vi "StrainTestCell3.vi"() -> ()   [LabVIEW 2020]
uses:
  <instrlib>/NH Research Regenerative Test Series/Public/Configure/Output Safety.ctl
  Readings.vi
  <instrlib>/NH Research Regenerative Test Series/Public/Data/Read (Ave Current).vi
  <instrlib>/NH Research Regenerative Test Series/Public/Data/Low Level/Fetch (Ave Voltage).vi
  <instrlib>/NH Research Regenerative Test Series/Public/Data/Low Level/Fetch (Ave True Power).vi
  <instrlib>/NH Research Regenerative Test Series/Public/Data/Read (Ave Voltage).vi
  <instrlib>/NH Research Regenerative Test Series/NH Research Regenerative Test Series.lvlib
panel:
  in  "Current Cutoff 2":dbl
  in  "Discharge Folder Path":path
  out "Charge Strain":dbl(graph)
  out "Discharge Strain":dbl(graph)
  in  "DWaitStop":bool
  out "Discharge Rest":bool
  in  "Wait Time":u32
  out "Elaspsed Time":u32 caption="Elapsed Time (s)"
  in  "CWait Stop":bool
  out "Charge Rest":bool
  in  "Wait Time":u32
  out "Elapsed Time":u32 caption="Elapsed Time (s)"
  out "Discharge Rest Voltage":dbl
  out "Charge Rest Voltage":dbl
  in  "1C Preset 2":bool
  out "Discharging":bool
  in  "Discharge Stop":bool
  in  "Discharge Current":dbl
  in  "Voltage Cutoff":dbl
  in  "1C Preset":bool
  out "Strain":dbl
  out "Ave Current (A)":dbl
  out "Ave Voltage (V)":dbl
  out "Ave True Power (W)":dbl
  out "Battemp":dbl
  out "AmbientTemp":dbl
  out "Discharge Rest Voltage":dbl(graph)
  out "Charge Rest Voltage":dbl(graph)
  in  "Tab Control":T1(tab)
  out "Selected Output Safety":T2
  in  "Custom Output Safety":T2
  in  "Output Safety\nSelection":bool caption="Output Safety"
  in  "Charge Folder Path":path
  in  "Cell Number":string
  in  "DAQmx Task Name":refnum<k21>
  in  "NHR VISA Name":refnum<visa-resource-name>
  out "Error Out":string
  out "Previous Discharge Data File":path caption="Filename Out"
  out "File Name":path caption="Filename Out"
  out "D Wait Status Byte Register":T3
  out "Discharge Status Byte Register":T3
  out "C Wait Status Byte Register":T3
  out "Charge Status Byte Register":T3
  out "Task error out":errorcluster
  in  "Cycle Stop":bool
  out "Cycle Index":i32
  in  "Number of Cycles":i32
  out "Charging":bool
  in  "Charge Stop":bool
  in  "Current Cutoff":dbl
  in  "Charge Current":dbl format="%#.6g"
  in  "Charge Voltage":dbl format="%#.6g"
  out "Tab Control 2":T1(tab)
  in  "Logical Instrument Number":u32=1
  # "Readings"
  # "Cycle & Charge Profile Settings"
  # "Charging"
  # "Discharging"
  # "Post Charge\nRest"
  # "Post Discharge\nRest"
  # "Cycle\nInfo"
  # "Rest Voltage Charts"
  # "Output Safety Configuration"
  # "Test Name & Device Info"
  # "Error Indication"
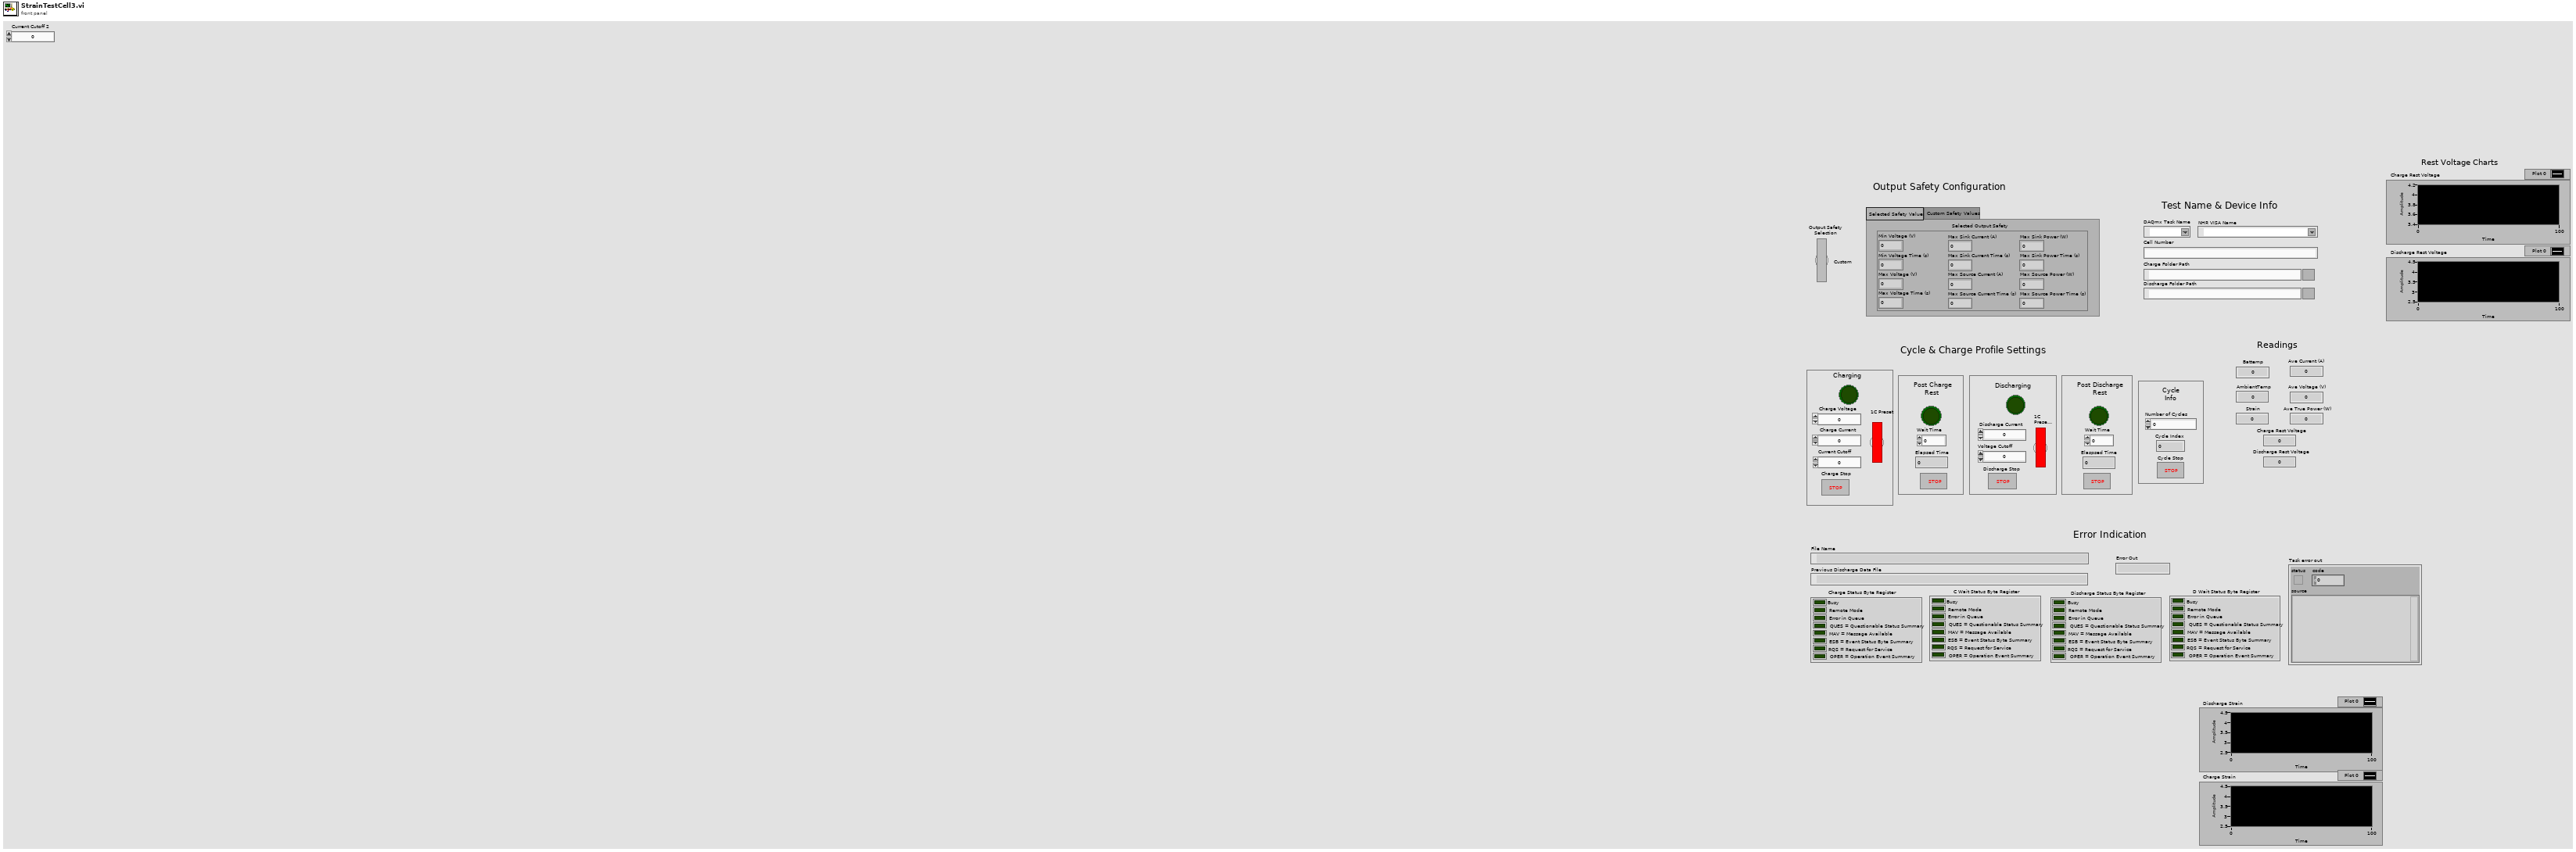
[diagram p1: front panel]
types:
  T1 = enum32{"Selected Safety Values", "Custom Safety Values"}
  T2 = typedef "NH Research Regenerative Test Series.lvlib/Output Safety.ctl" = cluster{"Min Voltage (V)":dbl, "Min Voltage Time (s)":dbl, "Max Voltage (V)":dbl, "Max Voltage Time (s)":dbl, "Max Sink Current (A)":dbl, "Max Sink Current Time (s)":dbl, "Max Source Current (A)":dbl, "Max Source Current Time (s)":dbl, "Max Sink Power (W)":dbl, "Max Sink Power Time (s)":dbl, "Max Source Power (W)":dbl, "Max Source Power Time (s)":dbl}
  T3 = cluster{"Busy":bool, "Remote Mode":bool, "Error in Queue":bool, "QUES = Questionable Status Summary":bool, "MAV = Message Available":bool, "ESB = Event Status Byte Summary":bool, "RQS = Request for Service":bool, "OPER = Operation Event Summary":bool}
  T4 = cluster{"Min Voltage (V)":dbl, "Min Voltage Time (s)":dbl, "Max Voltage (V)":dbl, "Max Voltage Time (s)":dbl, "Max Sink Current (A)":dbl, "Max Sink Current Time (s)":dbl, "Max Source Current (A)":dbl, "Max Source Current Time (s)":dbl, "Max Sink Power (W)":dbl, "Max Sink Power Time (s)":dbl, "Max Source Power (W)":dbl, "Max Source Power Time (s)":dbl}
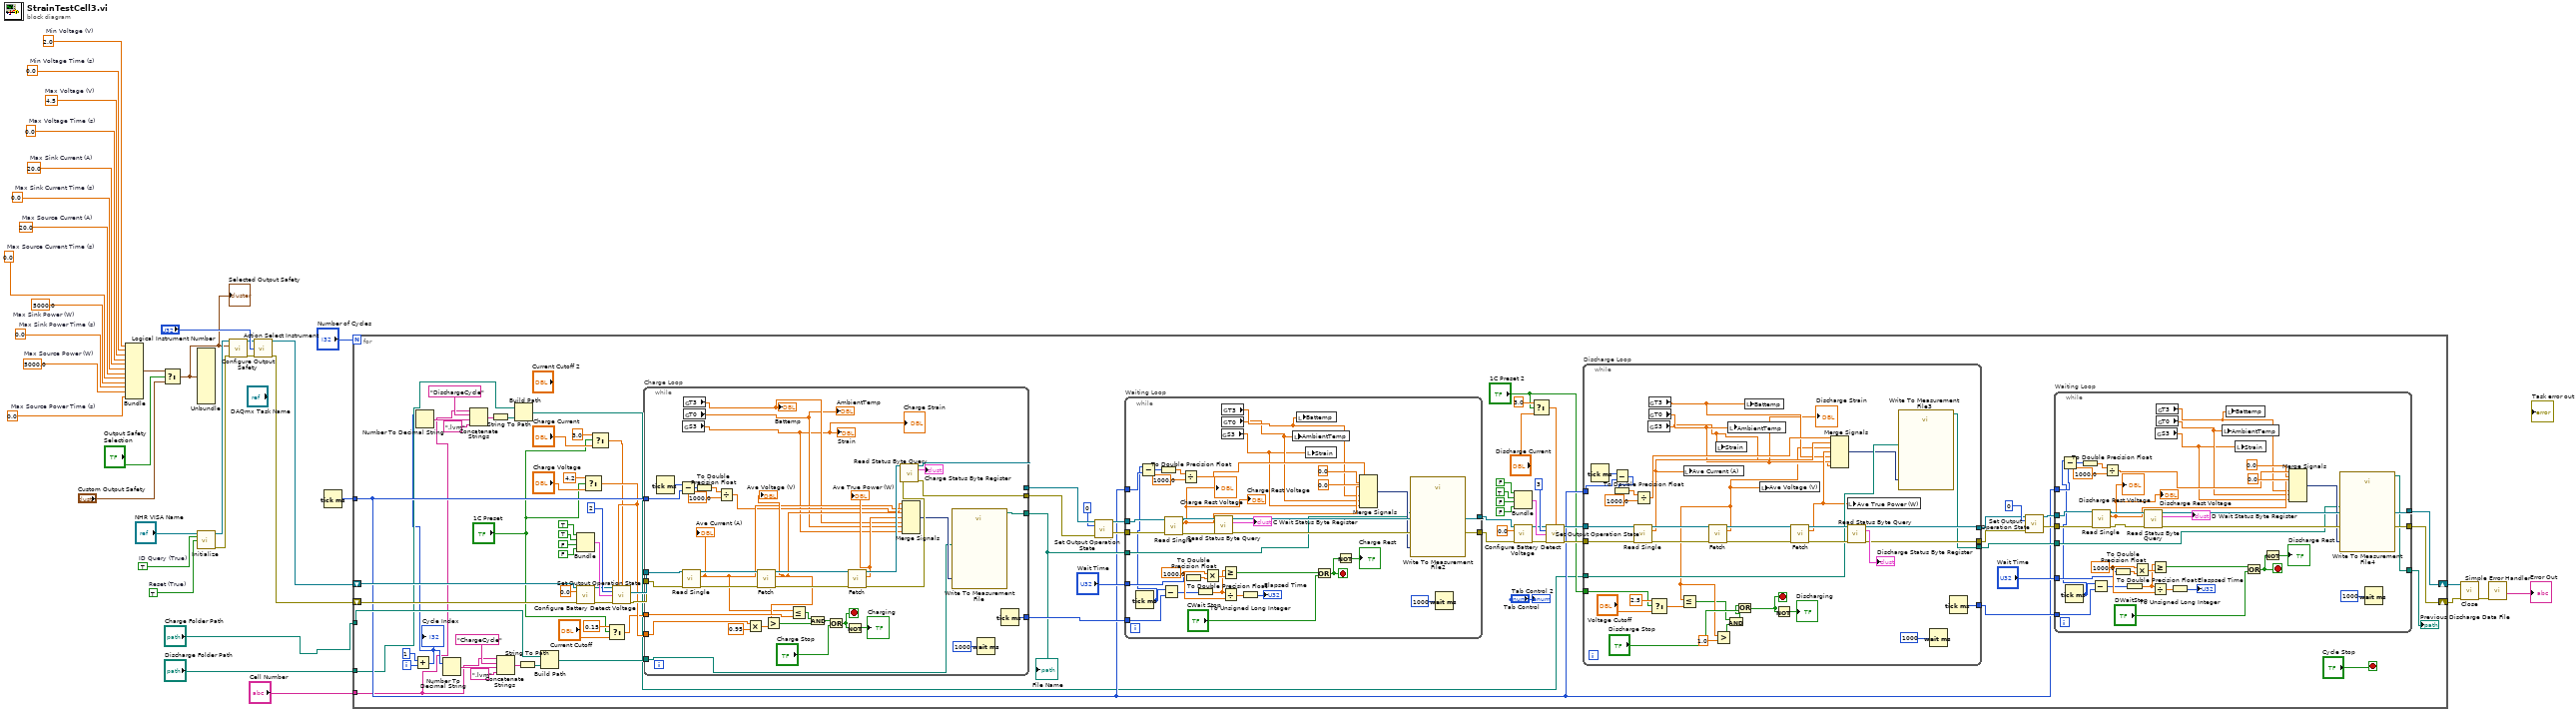
[diagram p0: block diagram]
diagram:
  w10 = 5000.0  # Max Source Power (W)
  w11 = 0.0  # Max Sink Power Time (s)
  w12 = 5000.0  # Max Sink Power (W)
  w13 = 0.0  # Max Source Current Time (s)
  w14 = 20.0  # Max Source Current (A)
  w16 = 20.0  # Max Sink Current (A)
  w15 = 0.0  # Max Sink Current Time (s)
  w17 = 0.0  # Max Voltage Time (s)
  w18 = 4.5  # Max Voltage (V)
  w19 = 2.0  # Min Voltage (V)
  w9 = 0.0  # Max Source Power Time (s)
  w20 = 0.0  # Min Voltage Time (s)
  w34 = TRUE  # ID Query (True)
  w33 = TRUE  # Reset (True)
  n1 = Bundle("Min Voltage (V)"=w19, "Min Voltage Time (s)"=w20, "Max Voltage (V)"=w18, "Max Voltage Time (s)"=w17, "Max Sink Current (A)"=w16, "Max Sink Current Time (s)"=w15, "Max Source Current (A)"=w14, "Max Source Current Time (s)"=w13, "Max Sink Power (W)"=w12, "Max Sink Power Time (s)"=w11, "Max Source Power (W)"=w10, "Max Source Power Time (s)"=w9) -> (w7:T4)  [unwired: 1 in]
  n2 = Select(t=w7, s="Output Safety\nSelection", f="Custom Output Safety") -> (s? t:f=w8:T2)
  "Selected Output Safety" <- w8
  n3 = Unbundle(w8) -> ()  [unwired: 12 out]
  n4 = call <vilib>:"Initialize.vi"("VISA resource name"="NHR VISA Name", "ID Query (True)"=w34, "Reset (True)"=w33) -> ("VISA resource name out"=w32:refnum<visa-resource-name>, "error out"=w31:errorcluster)  [unwired: 11 in]
  n5 = call <vilib>:"Configure Output Safety.vi"("VISA resource name"=w32, "Output Safety"=w8, "error in (no error)"=w31) -> ("VISA resource name out"=w29:refnum<visa-resource-name>, "error out"=w28:errorcluster)  [unwired: 11 in]
  n6 = call <instrlib>:"Action Select Instrument.vi"("VISA resource name"=w29, "Logical Instrument Number"="Logical Instrument Number", "error in (no error)"=w28) -> ("VISA resource name out"=w25:refnum<visa-resource-name>, "error out"=w24:errorcluster)  [unwired: 11 in]
  n7 = Tick Count (ms)() -> (millisecond timer value=w4:u32)
  n8 = for {
    N: "Number of Cycles" -> [_]
    shift-right: [w63] -> w23
    shift-left: w25 -> [w91]
    shift-right: [w62] -> w22
    shift-left: w24 -> [w89]
    tunnel: "Charge Folder Path" -> [w60]
    tunnel: w4 -> [w59]
    tunnel: "Cell Number" -> [w37]
    tunnel: "Discharge Folder Path" -> [w39]
    i -> [w86]
    stop <- "Cycle Stop" stop-if-true
    n9 = Add(x=1, y=w86) -> (x+y=w38:i32)
    "Cycle Index" <- w38
    n10 = Number To Decimal String(number=w38) -> (decimal integer string=w41:string)  [unwired: 1 in]
    n11 = Number To Decimal String(number=w38) -> (decimal integer string=w76:string)  [unwired: 1 in]
    n12 = Concatenate Strings(w37, "DischargeCycle", w41, ".lvm") -> (w42:string)
    n13 = String To Path(string=w42) -> (path=w43:path)
    n14 = Concatenate Strings(w37, "ChargeCycle", w76, ".lvm") -> (w81:string)
    n15 = Build Path(base path=w39, name or relative path=w43) -> (appended path=w36:path)
    n16 = String To Path(string=w81) -> (path=w82:path)
    n17 = Build Path(base path=w60, name or relative path=w82) -> (appended path=w78:path)
    n18 = Bundle(TRUE, TRUE, FALSE, FALSE) -> (w92:cluster{bool, bool, bool, bool})  [unwired: 1 in]
    n19 = call <vilib>:"Configure Battery Detect Voltage.vi"("VISA resource name"=w91, "Battery Detect Voltage (0V)"=0.0, "error in (no error)"=w89) -> ("VISA resource name out"=w90:refnum<visa-resource-name>, "error out"=w88:errorcluster)  [unwired: 11 in]
    n20 = Select(t=4.2, s="1C Preset", f="Charge Voltage") -> (s? t:f=w56:dbl)
    n21 = Select(t=3.0, s="1C Preset", f="Charge Current") -> (s? t:f=w55:dbl)
    n22 = Select(t=0.15, s="1C Preset", f="Current Cutoff") -> (s? t:f=w51:dbl)
    n23 = call <vilib>:"Set Output Operation State.vi"("VISA resource name"=w90, "Voltage Setpoint (0 V)"=w56, "Current Setpoint (0 A)"=w55, "Mode (0: Off)"=2, "Enable"=w92, "error in (no error)"=w88) -> ("VISA resource name out"=w98:refnum<visa-resource-name>, "error out"=w97:errorcluster)  [unwired: 8 in]
    n24 = while "Charge Loop" {
      tunnel: w98 -> [w257]
      tunnel: w97 -> [w256]
      tunnel: [w254] -> w103
      tunnel: [w253] -> w102
      tunnel: w51 -> [w249]
      tunnel: w78 -> [w244]
      tunnel: [w250] -> w72
      tunnel: [w245] -> w85
      tunnel: w56 -> [w236]
      tunnel: w59 -> [w234]
      stop <- w241 stop-if-true
      n25 = Tick Count (ms)() -> (millisecond timer value=w235:u32)
      n26 = Subtract(x=w235, y=w234) -> (x-y=w233:u32)
      n27 = call-poly <instrlib>:"Read Single.vi"("VISA resource name"=w257, "error in (no error)"=w256) -> ("VISA resource name out"=w262:refnum<visa-resource-name>, "Ave Current (A)"=w230:dbl, "error out"=w263:errorcluster)  [unwired: 11 in]
      "Ave Current (A)" <- w230
      n28 = global read "Readings.vi" "S3"() -> (w226:dbl)
      "Strain" <- w226
      "Charge Strain" <- w226
      n29 = global read "Readings.vi" "T3"() -> (w228:dbl)
      "Battemp" <- w228
      n30 = global read "Readings.vi" "T0"() -> (w227:dbl)
      "AmbientTemp" <- w227
      n31 = To Double Precision Float(number=w233) -> (double precision float=w231:dbl)
      n32 = Divide(x=w231, y=1000.0) -> (x/y=w229:dbl)
      n33 = Multiply(x=w236, y=0.95) -> (x*y=w238:dbl)
      n34 = call-poly <instrlib>:"Fetch.vi"("VISA resource name"=w262, "error in (no error)"=w263) -> ("VISA resource name out"=w261:refnum<visa-resource-name>, "Ave Voltage (V)"=w239:dbl, "error out"=w260:errorcluster)  [unwired: 11 in]
      "Ave Voltage (V)" <- w239
      n35 = Greater?(x=w239, y=w238) -> (0:w246:bool)
      n36 = Less Or Equal?(x=w230, y=w249) -> (x <= y?=w247:bool)
      n37 = And(x=w247, y=w246) -> (x .and. y?=w243:bool)
      n38 = Or(x=w243, y="Charge Stop") -> (x .or. y?=w241:bool)
      n39 = Not(x=w241) -> (.not. x?=→"Charging":bool)
      n40 = call-poly <instrlib>:"Fetch.vi"("VISA resource name"=w261, "error in (no error)"=w260) -> ("VISA resource name out"=w259:refnum<visa-resource-name>, "Ave True Power (W)"=w252:dbl, "error out"=w258:errorcluster)  [unwired: 11 in]
      "Ave True Power (W)" <- w252
      n41 = call <instrlib>:"Read Status Byte Query.vi"("VISA resource name"=w259, "error in (no error)"=w258) -> ("VISA resource name out"=w254:refnum<visa-resource-name>, "Status Byte Register"=→"Charge Status Byte Register":T3, "error out"=w253:errorcluster)  [unwired: 11 in]
      n42 = Merge Signals "Merge Signals"(w229, w230, w239, w252, w228, w227, w226) -> (w251:dynamicdata)
      n43 = call "Write To Measurement File"("Signals"=w251, "Filename"=w244) -> ("Filename Out"=w250:path)  [unwired: 15 in, 2 out]
      n44 = Wait (ms)(milliseconds to wait=u32 1000) -> ()  [unwired: 1 out]
      n45 = Tick Count (ms)() -> (millisecond timer value=w245:u32)
    }
    "File Name" <- w72
    n46 = call <vilib>:"Set Output Operation State.vi"("VISA resource name"=w103, "Mode (0: Off)"=0, "error in (no error)"=w102) -> ("VISA resource name out"=w100:refnum<visa-resource-name>, "error out"=w74:errorcluster)  [unwired: 11 in]
    n47 = while "Waiting Loop" {
      tunnel: [w224] -> w105
      tunnel: "Wait Time" -> [w214]
      tunnel: w85 -> [w221]
      tunnel: w100 -> [w205]
      tunnel: w74 -> [w204]
      tunnel: [w212] -> w73
      tunnel: w72 -> [w209]
      tunnel: w59 -> [w203]
      stop <- w194 stop-if-true
      w222 = 1000.0
      n48 = Tick Count (ms)() -> (millisecond timer value=w202:u32)
      n49 = Subtract(x=w202, y=w203) -> (x-y=w199:u32)
      n50 = To Double Precision Float(number=w199) -> (double precision float=w200:dbl)
      n51 = Subtract(x=w202, y=w221) -> (x-y=w216:u32)
      n52 = call-poly <instrlib>:"Read Single.vi"("VISA resource name"=w205, "error in (no error)"=w204) -> ("VISA resource name out"=w207:refnum<visa-resource-name>, "Ave Voltage (V)"=w206:dbl, "error out"=w208:errorcluster)  [unwired: 11 in]
      "Charge Rest Voltage" <- w206
      "Charge Rest Voltage" <- w206
      n53 = Divide(x=w200, y=1000.0) -> (x/y=w197:dbl)
      n54 = To Double Precision Float(number=w214) -> (double precision float=w213:dbl)
      n55 = To Double Precision Float(number=w216) -> (double precision float=w215:dbl)
      n56 = Multiply(x=w222, y=w213) -> (x*y=w223:dbl)
      n57 = call <instrlib>:"Read Status Byte Query.vi"("VISA resource name"=w207, "error in (no error)"=w208) -> ("VISA resource name out"=w224:refnum<visa-resource-name>, "Status Byte Register"=→"C Wait Status Byte Register":T3, "error out"=w212:errorcluster)  [unwired: 11 in]
      n58 = global read "Readings.vi" "S3"() -> (w191:dbl)
      n59 = global read "Readings.vi" "T3"() -> (w193:dbl)
      n60 = global read "Readings.vi" "T0"() -> (w192:dbl)
      n61 = Greater Or Equal?(x=w215, y=w223) -> (x >= y?=w196:bool)
      n62 = Divide(x=w215, y=w222) -> (x/y=w218:dbl)
      n63 = To Unsigned Long Integer(number=w218) -> (unsigned 32bit integer=→"Elapsed Time":u32)
      n64 = local write "AmbientTemp"(w192) -> ()
      n65 = local write "Battemp"(w193) -> ()
      n66 = local write "Strain"(w191) -> ()
      n67 = Or(x=w196, y="CWait Stop") -> (x .or. y?=w194:bool)
      n68 = Not(x=w194) -> (.not. x?=→"Charge Rest":bool)
      n69 = Merge Signals "Merge Signals"(w197, 0.0, w206, 0.0, w193, w192, w191) -> (w210:dynamicdata)
      n70 = call "Write To Measurement File2"("Signals"=w210, "Filename"=w209) -> ()  [unwired: 15 in, 3 out]
      n71 = Wait (ms)(milliseconds to wait=u32 1000) -> ()  [unwired: 1 out]
    }
    n72 = Bundle(FALSE, TRUE, FALSE, FALSE) -> (w107:cluster{bool, bool, bool, bool})  [unwired: 1 in]
    n73 = call <vilib>:"Configure Battery Detect Voltage.vi"("VISA resource name"=w105, "Battery Detect Voltage (0V)"=0.0, "error in (no error)"=w73) -> ("VISA resource name out"=w104:refnum<visa-resource-name>, "error out"=w106:errorcluster)  [unwired: 11 in]
    n74 = Select(t=3.0, s="1C Preset 2", f="Discharge Current") -> (s? t:f=w46:dbl)
    n75 = call <vilib>:"Set Output Operation State.vi"("VISA resource name"=w104, "Current Setpoint (0 A)"=w46, "Mode (0: Off)"=3, "Enable"=w107, "error in (no error)"=w106) -> ("VISA resource name out"=w112:refnum<visa-resource-name>, "error out"=w113:errorcluster)  [unwired: 9 in]
    n76 = while "Discharge Loop" {
      tunnel: w112 -> [w184]
      tunnel: w113 -> [w183]
      tunnel: [w181] -> w67
      tunnel: [w180] -> w68
      tunnel: w36 -> [w179]
      tunnel: [w169] -> w66
      tunnel: [w172] -> w65
      tunnel: w59 -> [w170]
      tunnel: "1C Preset 2" -> [w160]
      stop <- w174 stop-if-true
      n77 = Tick Count (ms)() -> (millisecond timer value=w171:u32)
      n78 = Subtract(x=w171, y=w170) -> (x-y=w166:u32)
      n79 = To Double Precision Float(number=w166) -> (double precision float=w167:dbl)
      n80 = call-poly <instrlib>:"Read Single.vi"("VISA resource name"=w184, "error in (no error)"=w183) -> ("VISA resource name out"=w189:refnum<visa-resource-name>, "Ave Current (A)"=w165:dbl, "error out"=w190:errorcluster)  [unwired: 11 in]
      n81 = Divide(x=w167, y=1000.0) -> (x/y=w164:dbl)
      n82 = global read "Readings.vi" "S3"() -> (w157:dbl)
      "Discharge Strain" <- w157
      n83 = global read "Readings.vi" "T3"() -> (w159:dbl)
      n84 = global read "Readings.vi" "T0"() -> (w158:dbl)
      n85 = Select(t=2.5, s=w160, f="Voltage Cutoff") -> (s? t:f=w161:dbl)
      n86 = local write "Ave Current (A)"(w165) -> ()
      n87 = call-poly <instrlib>:"Fetch.vi"("VISA resource name"=w189, "error in (no error)"=w190) -> ("VISA resource name out"=w188:refnum<visa-resource-name>, "Ave Voltage (V)"=w155:dbl, "error out"=w187:errorcluster)  [unwired: 11 in]
      n88 = Less Or Equal?(x=w155, y=w161) -> (x <= y?=w152:bool)
      n89 = Greater?(x=w155, y=1.0) -> (0:w154:bool)
      n90 = local write "Strain"(w157) -> ()
      n91 = And(x=w152, y=w154) -> (x .and. y?=w153:bool)
      n92 = local write "AmbientTemp"(w158) -> ()
      n93 = Or(x=w153, y="Discharge Stop") -> (x .or. y?=w174:bool)
      n94 = local write "Battemp"(w159) -> ()
      n95 = local write "Ave Voltage (V)"(w155) -> ()
      n96 = Not(x=w174) -> (.not. x?=→"Discharging":bool)
      n97 = call-poly <instrlib>:"Fetch.vi"("VISA resource name"=w188, "error in (no error)"=w187) -> ("VISA resource name out"=w186:refnum<visa-resource-name>, "Ave True Power (W)"=w173:dbl, "error out"=w185:errorcluster)  [unwired: 11 in]
      n98 = Merge Signals "Merge Signals"(w164, w165, w155, w173, w159, w158, w157) -> (w178:dynamicdata)
      n99 = local write "Ave True Power (W)"(w173) -> ()
      n100 = call <instrlib>:"Read Status Byte Query.vi"("VISA resource name"=w186, "error in (no error)"=w185) -> ("VISA resource name out"=w181:refnum<visa-resource-name>, "Status Byte Register"=→"Discharge Status Byte Register":T3, "error out"=w180:errorcluster)  [unwired: 11 in]
      n101 = call "Write To Measurement File3"("Signals"=w178, "Filename"=w179) -> ("Filename Out"=w172:path)  [unwired: 15 in, 2 out]
      n102 = Wait (ms)(milliseconds to wait=u32 1000) -> ()  [unwired: 1 out]
      n103 = Tick Count (ms)() -> (millisecond timer value=w169:u32)
    }
    n104 = call <vilib>:"Set Output Operation State.vi"("VISA resource name"=w67, "Mode (0: Off)"=0, "error in (no error)"=w68) -> ("VISA resource name out"=w71:refnum<visa-resource-name>, "error out"=w70:errorcluster)  [unwired: 11 in]
    n105 = while "Waiting Loop" {
      tunnel: [w151] -> w63
      tunnel: "Wait Time" -> [w143]
      tunnel: w66 -> [w148]
      tunnel: w71 -> [w133]
      tunnel: w70 -> [w132]
      tunnel: [w141] -> w62
      tunnel: [w138] -> w61
      tunnel: w65 -> [w137]
      tunnel: w59 -> [w128]
      stop <- w119 stop-if-true
      w149 = 1000.0
      n106 = Tick Count (ms)() -> (millisecond timer value=w127:u32)
      n107 = Subtract(x=w127, y=w128) -> (x-y=w124:u32)
      n108 = To Double Precision Float(number=w124) -> (double precision float=w125:dbl)
      n109 = Subtract(x=w127, y=w148) -> (x-y=w145:u32)
      n110 = call-poly <instrlib>:"Read Single.vi"("VISA resource name"=w133, "error in (no error)"=w132) -> ("VISA resource name out"=w131:refnum<visa-resource-name>, "Ave Voltage (V)"=w130:dbl, "error out"=w129:errorcluster)  [unwired: 11 in]
      "Discharge Rest Voltage" <- w130
      "Discharge Rest Voltage" <- w130
      n111 = Divide(x=w125, y=1000.0) -> (x/y=w123:dbl)
      n112 = To Double Precision Float(number=w143) -> (double precision float=w142:dbl)
      n113 = To Double Precision Float(number=w145) -> (double precision float=w144:dbl)
      n114 = Multiply(x=w149, y=w142) -> (x*y=w150:dbl)
      n115 = call <instrlib>:"Read Status Byte Query.vi"("VISA resource name"=w131, "error in (no error)"=w129) -> ("VISA resource name out"=w151:refnum<visa-resource-name>, "Status Byte Register"=→"D Wait Status Byte Register":T3, "error out"=w141:errorcluster)  [unwired: 11 in]
      n116 = Greater Or Equal?(x=w144, y=w150) -> (x >= y?=w121:bool)
      n117 = Divide(x=w144, y=w149) -> (x/y=w146:dbl)
      n118 = global read "Readings.vi" "S3"() -> (w116:dbl)
      n119 = global read "Readings.vi" "T3"() -> (w118:dbl)
      n120 = global read "Readings.vi" "T0"() -> (w117:dbl)
      n121 = To Unsigned Long Integer(number=w146) -> (unsigned 32bit integer=→"Elaspsed Time":u32)
      n122 = local write "AmbientTemp"(w117) -> ()
      n123 = local write "Battemp"(w118) -> ()
      n124 = local write "Strain"(w116) -> ()
      n125 = Or(x=w121, y="DWaitStop") -> (x .or. y?=w119:bool)
      n126 = Not(x=w119) -> (.not. x?=→"Discharge Rest":bool)
      n127 = Merge Signals "Merge Signals"(w123, 0.0, w130, 0.0, w118, w117, w116) -> (w139:dynamicdata)
      n128 = call "Write To Measurement File4"("Signals"=w139, "Filename"=w137) -> ("Filename Out"=w138:path)  [unwired: 15 in, 2 out]
      n129 = Wait (ms)(milliseconds to wait=u32 1000) -> ()  [unwired: 1 out]
    }
    "Previous Discharge Data File" <- w61
    "Tab Control 2" <- "Tab Control"
  }
  n130 = call <instrlib>:"Close.vi"("VISA resource name"=w23, "error in (no error)"=w22) -> ("error out"=w27:errorcluster)  [unwired: 13 in]
  n131 = call <vilib>:"Simple Error Handler.vi"("error in (no error)"=w27) -> ("source out"=→"Error Out":string)  [unwired: 4 in, 4 out]
